vi "MPM_Get_Mode_Information.vi"(8 "error in (no error)":errorcluster, 10 "moduleNumber":i32, 11 ".NET Reference in":refnum<k24>) -> (0 "error out":errorcluster, 2 "info":string, 3 "Reference out":refnum<k24>)   [LabVIEW 2017]
uses:
  LV_IL_Sample/DLL/InstrumentDLL.dll
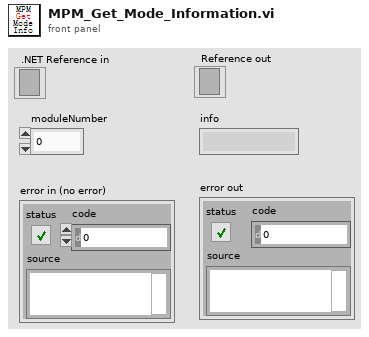
[diagram p1: front panel]
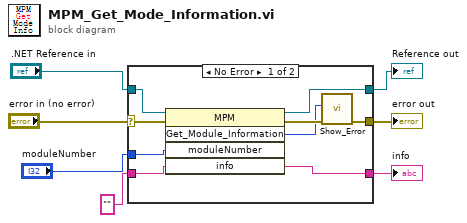
[diagram p0: block diagram]
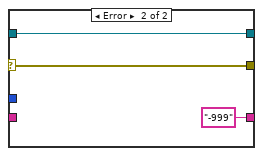
[diagram p2: hidden frame]
diagram:
  n1 = case shown="No Error" "error in (no error)" {
    selector: "error in (no error)" -> [w14 w18]
    tunnel: ".NET Reference in" -> [w16 w19]
    tunnel: [w15 w19] -> w6
    tunnel: [w13 w18] -> w4
    tunnel: "moduleNumber" -> [w10 _]
    tunnel: "" ("info") -> [w9 _]
    tunnel: [w8 "-999" ("info")] -> w1
    frame No Error {
      n2 = invoke class="MPM" method="Get_Module_Information"(reference=w16, error in=w14, "moduleNumber"=w10, "info"=w9) -> (reference out=w15:refnum<k24>, error out=w12:errorcluster, "Get_Module_Information"=w11:i32, "info"=w8:string)  [unwired: 1 in, 1 out]
      n3 = call "Show_Error.vi"("error in (no error)"=w12, "Error"=w11) -> ("error out"=w13:errorcluster)  [unwired: 9 in]
    }
    frame Error {
    }
  }
  "Reference out" <- w6
  "error out" <- w4
  "info" <- w1
